vi "CRYGet Protected Stimulus.vi"(11 "Name":string) -> (3 "Protect Names":string[](array[string]))   [LabVIEW 2013]
uses:
  Global/CRYCurves Array Global.vi
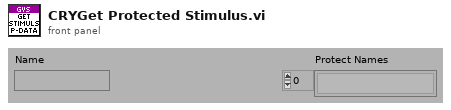
[diagram p1: front panel]
types:
  T1 = typedef "CRYWaveform Cluster Array.ctl" = T2[]
  T2 = typedef "CRYWaveform Cluster.ctl" = cluster{"Waveform":cluster{"X0":dbl, "dX":dbl, "Y":sgl[]}, "X data":u16, "Y data":u16, "Y axis":u16, "X unit":string, "Y unit":string, "Y dB ref":dbl, "display Y":bool, "display X":bool, "Overload?":bool, "Test Info":string, "Step No.":i32, "Name":string, "protected":bool, "Sqc history":string[], "Signal Channel ID":i32, "Plot Settings":cluster{"Color":u32, "Interpolation":u8, "Point Style":u8, "Line Style":u8, "Point Color":u32, "Line Width":u8, "Bar Plot Style":u8, "Fill To":i16}, "AutoProtect":bool}
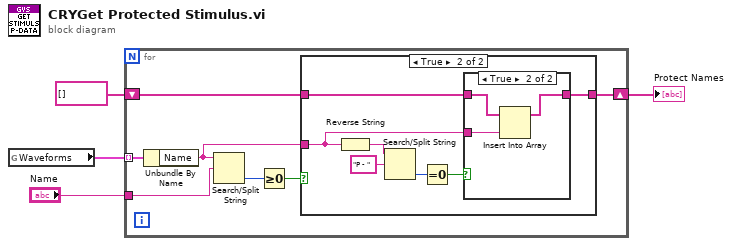
[diagram p0: block diagram]
diagram:
  n1 = global read "CRYCurves Array Global.vi" "Waveforms"() -> (w1:T1)
  n2 = for {
    shift-right: [w9] -> w3
    shift-left: string[] [] ("Protect Names") -> [w10]
    tunnel: w1 -> [w11] mode=indexing
    tunnel: "Name" -> [w8]
    n3 = Unbundle By Name(w11) -> ("Name"=w5:string)
    n4 = Search/Split String(string=w5, search string/char (-)=w8) -> (offset of match=w7:i32)  [unwired: 3 out]
    n5 = Greater Or Equal To 0?(x=w7) -> (x >= 0?=w6:bool)
    n6 = case shown="True" w6 {
      tunnel: w10 -> [w12 w15]
      tunnel: [w12 w14] -> w9
      tunnel: w5 -> [_ w13]
      frame False {
      }
      frame True {
        n7 = Reverse String(1:w13) -> (0:w17:string)
        n8 = Search/Split String(string=w17, search string/char (-)="P - ") -> (offset of match=w18:i32)  [unwired: 3 out]
        n9 = Equal To 0?(x=w18) -> (x = 0?=w16:bool)
        n10 = case shown="True" w16 {
          tunnel: [w20 w22] -> w14
          tunnel: w15 -> [w20 w23]
          tunnel: w13 -> [_ w21]
          frame False {
          }
          frame True {
            n11 = Insert Into Array(array=w23, new element=w21) -> (w22:string[])  [unwired: 1 in]
          }
        }
      }
    }
  }
  "Protect Names" <- w3
